vi "SwerveModuleOdometry.vi"(4 "Robot Heading(deg)":dbl, 7 "Wheel Azimuth (deg)":dbl, 9 "Velocity (ft/s)":dbl) -> (0 "Delta Y (in)":dbl, 1 "Delta X (in)":dbl, 2 "Velocity Y (ft/s)":dbl, 3 "Velocity X (ft/s)":dbl)   [LabVIEW 2020]
doc: "This VI calculates the field-centric delta odometry and velocity vectors for a single swerve module."
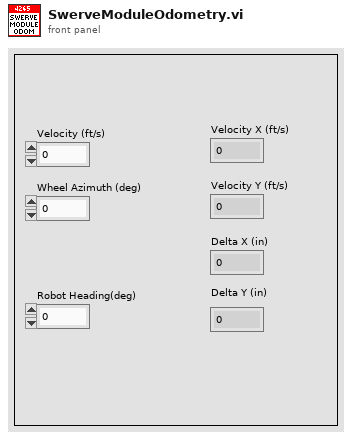
[diagram p1: front panel]
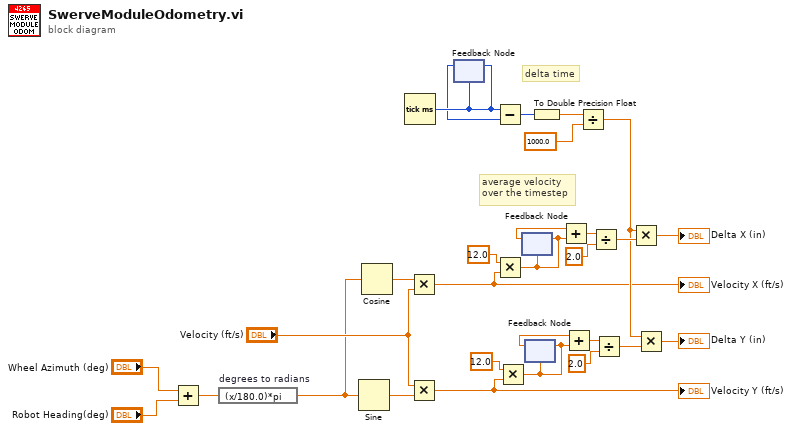
[diagram p0: block diagram]
diagram:
  # "delta time"
  # "average velocity\nover the timestep"
  n1 = Add(x="Wheel Azimuth (deg)", y="Robot Heading(deg)") -> (x+y=w27:dbl)
  n2 = expression code="(x/180.0)*pi" "degrees to radians"(w27) -> (w18:dbl)
  n3 = Sine(x=w18) -> (sin(x)=w26:dbl)
  n4 = Cosine(x=w18) -> (cos(x)=w25:dbl)
  n5 = Tick Count (ms)() -> (millisecond timer value=w24:u32)
  n6 = Multiply(x=w25, y="Velocity (ft/s)") -> (x*y=w2:dbl)
  "Velocity X (ft/s)" <- w2
  n7 = Multiply(x="Velocity (ft/s)", y=w26) -> (x*y=w1:dbl)
  "Velocity Y (ft/s)" <- w1
  n8 = feedback-in #1(w24) -> ()
  n9 = feedback #1(w24) -> (w23:u32)
  n10 = Subtract(x=w24, y=w23) -> (x-y=w22:u32)
  n11 = Multiply(x=12.0 ("y"), y=w2) -> (x*y=w14:dbl)
  n12 = Multiply(x=12.0 ("y"), y=w1) -> (x*y=w9:dbl)
  n13 = feedback #2(w14) -> (w13:dbl)
  n14 = feedback-in #2(w14) -> ()
  n15 = feedback #3(w9) -> (w8:dbl)
  n16 = feedback-in #3(w9) -> ()
  n17 = To Double Precision Float(number=w22) -> (double precision float=w21:dbl)
  n18 = Add(x=w13, y=w14) -> (x+y=w16:dbl)
  n19 = Add(x=w8, y=w9) -> (x+y=w11:dbl)
  n20 = Divide(x=w21, y=1000.0) -> (x/y=w5:dbl)
  n21 = Divide(x=w16, y=2.0) -> (x/y=w7:dbl)
  n22 = Divide(x=w11, y=2.0) -> (x/y=w6:dbl)
  n23 = Multiply(x=w5, y=w7) -> (x*y=→"Delta X (in)":dbl)
  n24 = Multiply(x=w5, y=w6) -> (x*y=→"Delta Y (in)":dbl)
